vi "get tree display name.vi"(8 "error in (no error)":errorcluster, 11 "TreeControl in":refnum<vi>) -> (0 "error out":errorcluster, 2 "display name":string, 3 "TreeControl out":refnum<vi>)   [LabVIEW 2017]
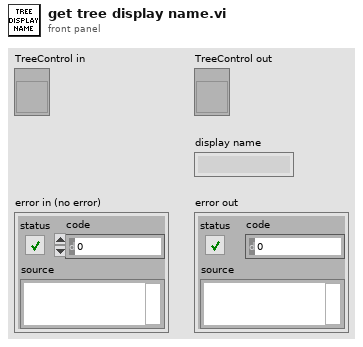
[diagram p1: front panel]
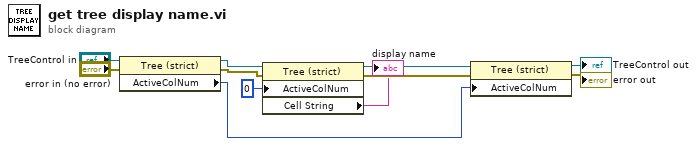
[diagram p0: block diagram]
diagram:
  n1 = property class="Tree (strict)"(reference="TreeControl in", error in="error in (no error)") -> (reference out=w3:refnum<vi>, error out=w6:errorcluster, "ActiveColNum"=w5:i32)
  n2 = property class="Tree (strict)"(reference=w3, error in=w6, "ActiveColNum"=0 ("Active Cell:Active Column Number")) -> (reference out=w4:refnum<vi>, error out=w7:errorcluster, "Cell String"=→"display name":string)
  n3 = property class="Tree (strict)"(reference=w4, error in=w7, "ActiveColNum"=w5) -> (reference out=→"TreeControl out":refnum<vi>, error out=→"error out":errorcluster)
